vi "XW_Tutu_Chevray_PN.vi"() -> (5 "Plug in titles":string[](array[string]), 7 "Plug in values":string[](array[string]))   [LabVIEW 2020]
uses:
  Globals/Meas_global.vi
  Controls/Analysis_type_Enum.ctl
  <vilib>/Utility/file.llb/Read From Spreadsheet File (string).vi
panel:
  out "UW":bool
  out "Converged":bool=TRUE
  out "Third":dbl format="%#.3f"
  out "Filename":string
  out "Third Component":path
  out "Info index":i32
  out "2nd Comp":string
  out "1st Comp":string
  out "Psi 2":dbl=-999.0 format="%.2f"
  out "Psi 1":dbl=-999.0 format="%.2f"
  out "Indicies":i32[](array[numeric])
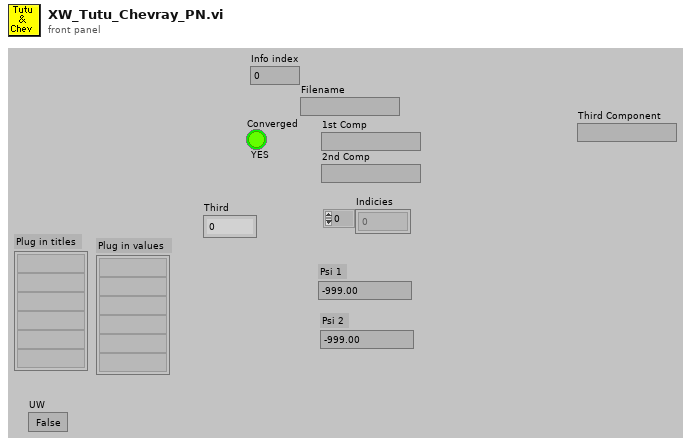
[diagram p1: front panel]
types:
  T1 = typedef "Correlation_cluster1.ctl" = cluster{"U inst":string, "uw":dbl, "u^2w":dbl, "uw^2":dbl, "uw/u'w'":dbl, "W inst":string, "uw^3":dbl, "u^3w":dbl, "u^2w^2":dbl, "Index U":i32, "Index W":i32, "Error info":string[], "Paired Sampling Rate (Hz)":dbl, "u^2 Paired":dbl, "w^2 Paired":dbl, "Time Window (ms)":dbl}
  T2 = typedef "Analysis_info_cluster.ctl" = cluster{"Colour":u32, "Inst type":T3, "Inst name":string, "Symbol":string, "Code name":string, "Extra Info":string, "Inst Array":T4, "Extra Titles":string[], "Extra Values":string[], "U":dbl, "u^2":dbl, "u^3":dbl, "u^4":dbl, "Skew_u":dbl, "Kurt_u":dbl, "Sd Error in Mean":dbl, "% u'/U":dbl, "X":dbl, "Y":dbl, "Z":dbl, "Timescale integral Estimate":dbl, "Sd Error in Variance":dbl, "Calib File":path, "Calib Constants":dbl[], "Output Position":bool, "Stats":enum16{"None", "Basic", "Full"}, "Av Sampling Rate":dbl, "Av No of Samples":dbl, "Total Meas Time (s)":dbl, "ADAM Ch Name":string, "Max value":dbl, "Min value":dbl, "Req Sample Rate Hz":dbl, "Sync Delay Time (s)":dbl, "Ch No":i16, "Device":string, "Use Latest Calib":bool, "Port":string, "Metadata Ch Names":string[], "Metadata Ch Values":string[], "Label":string}
  T3 = typedef "Inst_type.ctl" = enum16{"Raw voltage", "Raw with zero offsetting", "Propeller anemometer", "Pressure Transducer", "Pitot-static tube", "Hot wire", "Cross wire 1", "Cross wire 2", "Generic Linear", "Generic Polynomial", "Generic BackPoly", "Fast FID", "Thermocouple", "Cold wire", "Pulsed Wire", "LDA Vel", "LDA Tran time", "LDA Arr time", "Microphone"}
  T4 = typedef "Instrument_Array.ctl" = enum16{"PWA", "LDA", "Analogue"}
  T5 = typedef "Analysis_type_Enum.ctl" = enum16{"Slow Response", "Fast Response", "Weighted Fast Response", "Fast FID", "Weighted Fast FID", "Cross Wire", "Weighted Cross Wire", "Weighted LDA"}
  T6 = enum16{"Save no data", "Save data in new files", "Save data in existing files"}
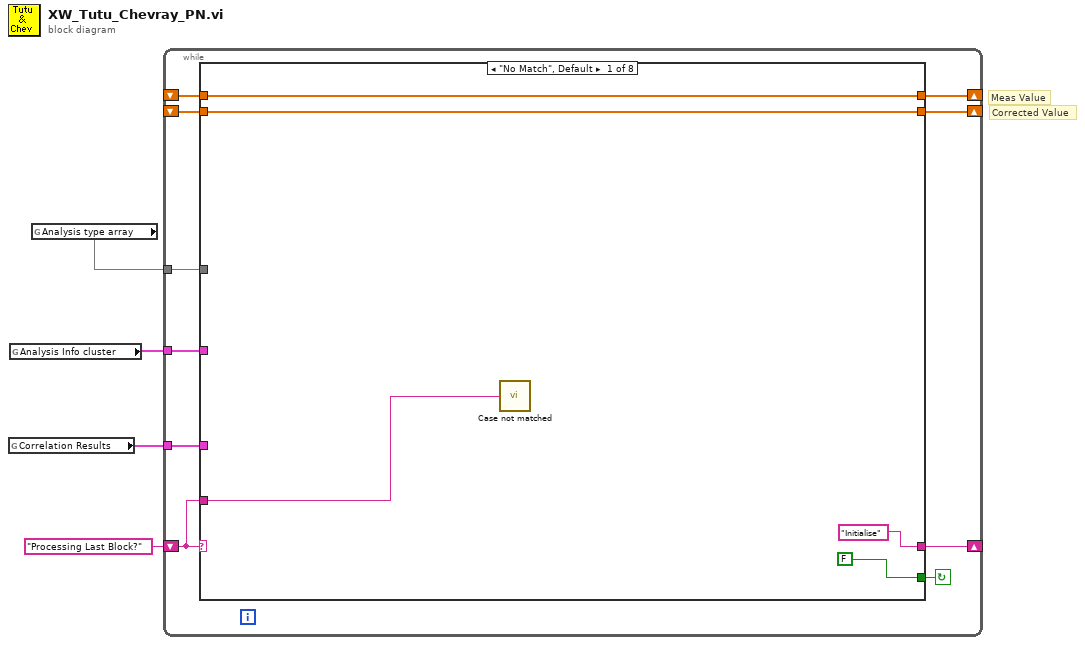
[diagram p0: block diagram]
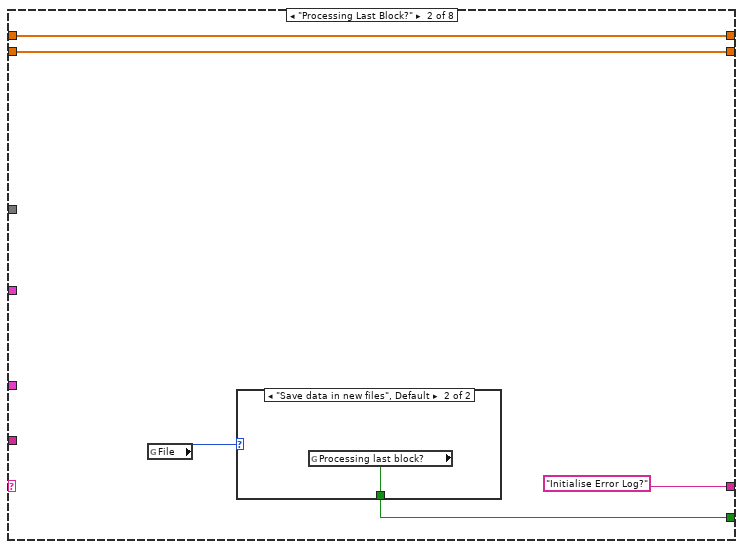
[diagram p2: hidden frame]
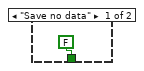
[diagram p3: hidden frame]
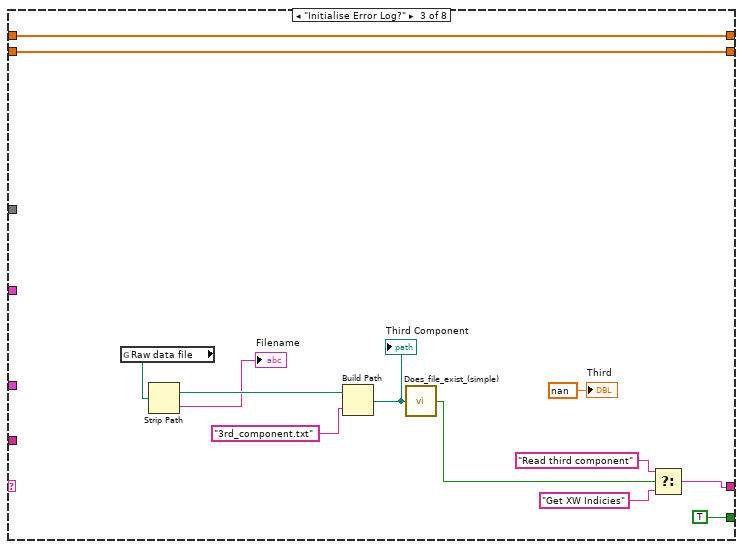
[diagram p4: hidden frame]
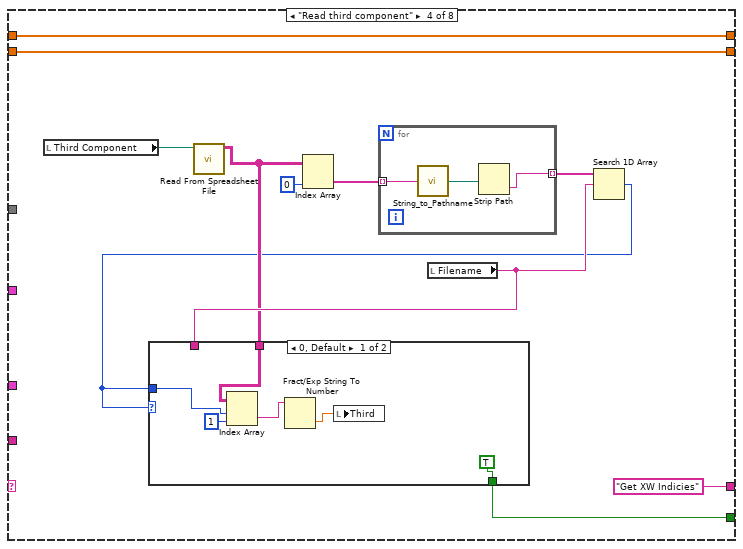
[diagram p5: hidden frame]
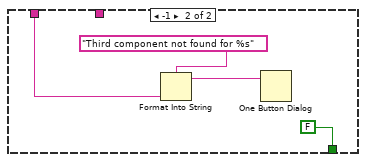
[diagram p6: hidden frame]
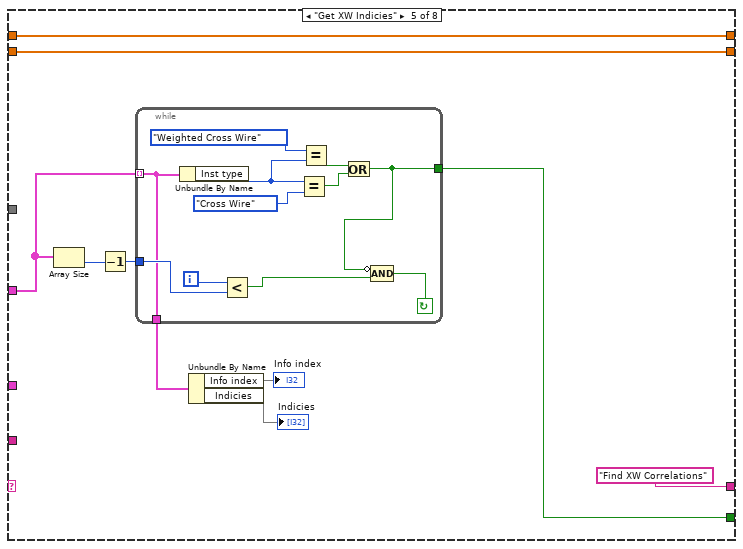
[diagram p7: hidden frame]
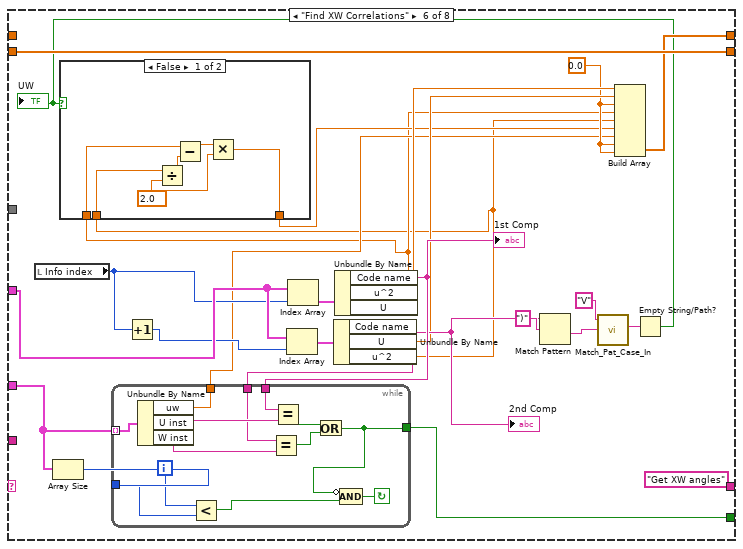
[diagram p8: hidden frame]
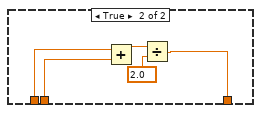
[diagram p9: hidden frame]
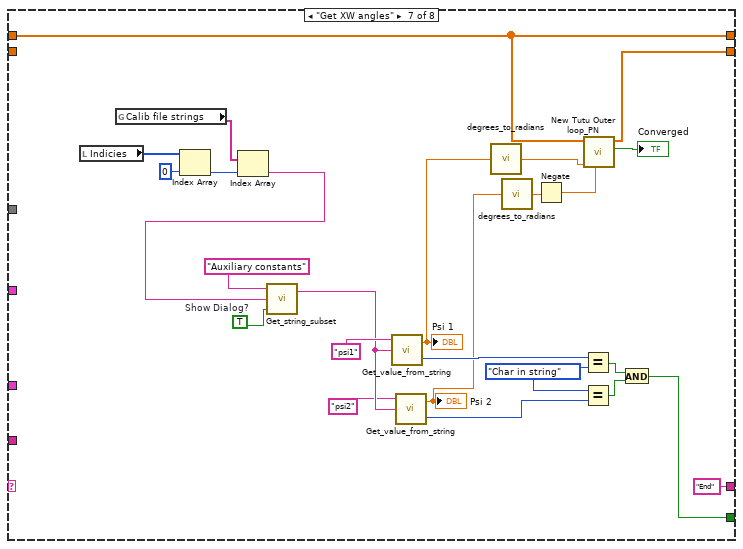
[diagram p10: hidden frame]
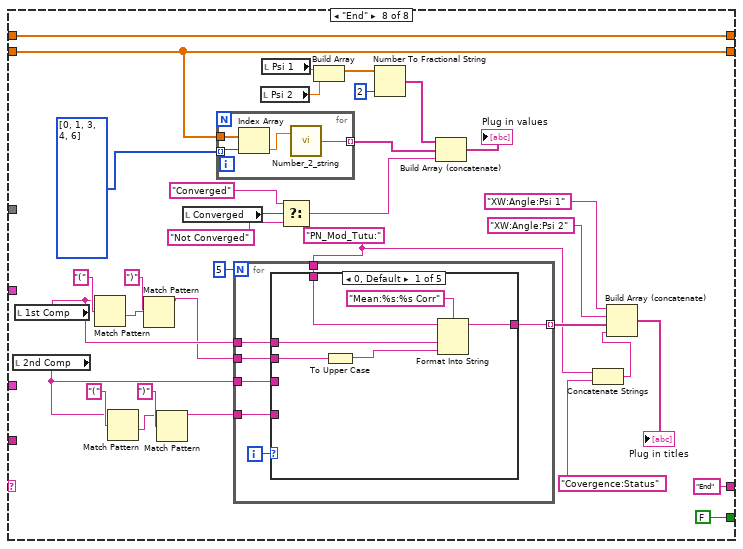
[diagram p11: hidden frame]
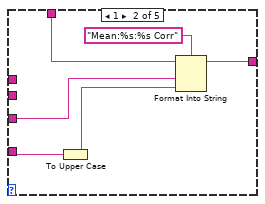
[diagram p12: hidden frame]
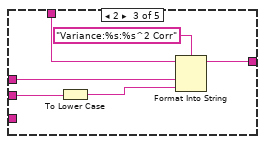
[diagram p13: hidden frame]
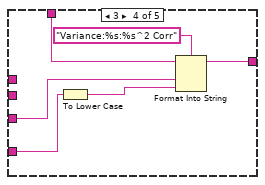
[diagram p14: hidden frame]
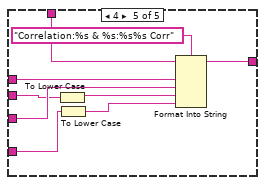
[diagram p15: hidden frame]
diagram:
  # "Corrected Value"
  # "Meas Value"
  n1 = global read "Meas_global.vi" "Correlation Results"() -> (w1:T1[])
  n2 = global read "Meas_global.vi" "Analysis Info cluster"() -> (w2:T2[])
  n3 = global read "Meas_global.vi" "Analysis type array"() -> (w3)
  n4 = while {
    tunnel: w1 -> [w6]
    tunnel: w2 -> [w7]
    tunnel: w3 -> [w11]
    shift-left: _ -> [w5]
    shift-right: [w8] -> _
    shift-left: _ -> [w9]
    shift-right: [w10] -> _
    shift-left: "Processing Last Block?" -> [w12]
    shift-right: [w13] -> _
    stop <- w14 continue-if-true
    n5 = case shown="\"No Match\", Default" w12 {
      tunnel: [FALSE w23 TRUE ("Processing last block?") w42 w69 w94 w142 FALSE ("Processing last block?")] -> w14
      tunnel: ["Initialise" "Initialise Error Log?" w29 "Get XW Indicies" "Find XW Correlations" "Get XW angles" "End" "End"] -> w13
      tunnel: w12 -> [w15 _ _ _ _ _ _ _]
      tunnel: w11 -> [_ _ _ _ _ _ _ _]
      tunnel: [w17 w22 w39 w50 w68 w96 w141 w190] -> w10
      tunnel: w9 -> [w17 w22 w39 w50 w68 _ w141 w190]
      tunnel: [w16 w20 w38 w49 w67 w108 w140 w166] -> w8
      tunnel: w7 -> [_ _ _ _ w64 w105 _ _]
      tunnel: w6 -> [_ _ _ _ _ w104 _ _]
      tunnel: w5 -> [w16 w20 w38 w49 w67 w108 _ w166]
      frame "No Match", Default {
        n6 = call "Case not matched.vi"("Case Name not Matched"=w15) -> ()
      }
      frame "Processing Last Block?" {
        n7 = global read "Meas_global.vi" "File"() -> (w21:T6)
        n8 = case shown="\"Save data in new files\", Default" w21 {
          tunnel: [FALSE ("Processing last block?") w26] -> w23
          frame "Save no data" {
          }
          frame "Save data in new files", Default {
            n9 = global read "Meas_global.vi" "Processing last block?"() -> (w26:bool)
          }
        }
      }
      frame "Initialise Error Log?" {
        n10 = global read "Meas_global.vi" "Raw data file"() -> (w36:path)
        n11 = Strip Path(path=w36) -> (stripped path=w35:path, name=→"Filename":string)
        n12 = Build Path(base path=w35, name or relative path="3rd_component.txt") -> (appended path=w33:path)
        "Third Component" <- w33
        n13 = call "Does_file_exist_(simple).vi"("Pathname"=w33) -> ("exists?"=w30:bool)
        n14 = Select(t="Read third component", s=w30, f="Get XW Indicies") -> (s? t:f=w29:string)
        "Third" <- nan ("Third")
      }
      frame "Read third component" {
        n15 = local read "Third Component"() -> (w47:path)
        n16 = call-poly <vilib>:"Read From Spreadsheet File.vi"("file path (dialog if empty)"=w47) -> ("all rows"=w41:string[][])  [unwired: 3 in, 7 out]
        n17 = Index Array(array=w41, index (col)=0 ("disabled index (col)")) -> (element=w45:string[])  [unwired: 1 in]
        n18 = for {
          tunnel: w45 -> [w63] mode=indexing
          tunnel: [w61] -> w44 mode=indexing
          n19 = call "String_to_Pathname.vi"("Input String"=w63) -> ("path"=w62:path)
          n20 = Strip Path(path=w62) -> (name=w61:string)  [unwired: 1 out]
        }
        n21 = local read "Filename"() -> (w43:string)
        n22 = Search 1D Array(1D array=w44, element=w43) -> (index of element=w40:i32)  [unwired: 1 out]
        n23 = case shown="0, Default" w40 {
          tunnel: w43 -> [_ w60]
          tunnel: [TRUE ("Processing last block?") FALSE ("Processing last block?")] -> w42
          tunnel: w41 -> [w54 _]
          tunnel: w40 -> [w53 _]
          frame 0, Default {
            n24 = Index Array(array=w54, index (row)=w53, index (col)=1 ("disabled index (col)")) -> (element=w52:string)
            n25 = Fract/Exp String To Number(string=w52) -> (number=w51:dbl)  [unwired: 4 out]
            n26 = local write "Third"(w51) -> ()
          }
          frame -1 {
            n27 = Format Into String(format string="Third component not found for %s" ("message"), w60) -> (resulting string=w58:string)  [unwired: 2 in, 1 out]
            n28 = One Button Dialog(message=w58) -> ()  [unwired: 2 out]
          }
        }
      }
      frame "Get XW Indicies" {
        n29 = Array Size(array=w64) -> (size(s)=w72:i32)
        n30 = Decrement(x=w72) -> (x-1=w71:i32)
        n31 = while {
          tunnel: [w74] -> w69
          tunnel: [w75] -> w70
          tunnel: w71 -> [w78]
          tunnel: w64 -> [w75] mode=indexing
          i -> [w79]
          stop <- w76 continue-if-true
          n32 = Unbundle By Name(w75) -> ("Inst type"=w83:T3)
          n33 = Less?(x=w79, y=w78) -> (x < y?=w77:bool)
          n34 = Equal?(x=w83, y=Analysis_type_Enum."Cross Wire" ("Analysis type")) -> (x = y?=w81:bool)
          n35 = Equal?(x=Analysis_type_Enum."Weighted Cross Wire" ("Analysis type"), y=w83) -> (x = y?=w80:bool)
          n36 = Or(x=w80, y=w81) -> (x .or. y?=w74:bool)
          n37 = Compound Arithmetic op=AND(invert w74, w77) -> (w76:bool)
        }
        n38 = Unbundle By Name(w70) -> ("Info index"=→"Info index", "Indicies"=→"Indicies")
      }
      frame "Find XW Correlations" {
        w90 = 0.0 ("element")
        n39 = local read "Info index"() -> (w93:i32)
        n40 = Array Size(array=w104) -> (size(s)=w102:i32)
        n41 = Increment(x=w93) -> (x+1=w92:i32)
        n42 = Index Array(array=w105, index=w92) -> (element=w106:T2)
        n43 = Index Array(array=w105, index=w93) -> (element=w107:T2)
        n44 = Unbundle By Name(w106) -> ("Code name"=w100:string, "U"=w91:dbl, "u^2"=w86:dbl)
        "2nd Comp" <- w100
        n45 = Unbundle By Name(w107) -> ("Code name"=w103:string, "u^2"=w87:dbl, "U"=w95:dbl)
        "1st Comp" <- w103
        n46 = while {
          tunnel: [w121] -> w89
          tunnel: w100 -> [w122]
          tunnel: w103 -> [w123]
          tunnel: w104 -> [w126] mode=indexing
          tunnel: [w127] -> w94
          tunnel: w102 -> [w130]
          i -> [w131]
          stop <- w128 continue-if-true
          n47 = Unbundle By Name(w126) -> ("uw"=w121:dbl, "U inst"=w125:string, "W inst"=w124:string)
          n48 = Less?(x=w131, y=w130) -> (x < y?=w129:bool)
          n49 = Equal?(x=w122, y=w124) -> (x = y?=w133:bool)
          n50 = Equal?(x=w123, y=w125) -> (x = y?=w132:bool)
          n51 = Or(x=w132, y=w133) -> (x .or. y?=w127:bool)
          n52 = Compound Arithmetic op=AND(invert w127, w129) -> (w128:bool)
        }
        n53 = Match Pattern(string=w100, regular expression=")") -> (after substring=w98:string)  [unwired: 4 out]
        n54 = call "Match_Pat_Case_In.vi"("String to match"="V" ("regular expression"), "String"=w98) -> ("Matched string"=w97:string)  [unwired: 1 in, 3 out]
        n55 = Empty String/Path?(string/path=w97) -> (empty?=w85:bool)
        "UW" <- w85
        n56 = case shown="False" w85 {
          tunnel: w87 -> [w111 w117]
          tunnel: w86 -> [w110 w116]
          tunnel: [w112 w118] -> w88
          frame False {
            w113 = 2.0 ("y")
            n57 = Divide(x=w110, y=w113) -> (x/y=w115:dbl)
            n58 = Subtract(x=w111, y=w115) -> (x-y=w114:dbl)
            n59 = Multiply(x=w114, y=w113) -> (x*y=w112:dbl)
          }
          frame True {
            n60 = Add(x=w117, y=w116) -> (x+y=w120:dbl)
            n61 = Divide(x=w120, y=2.0) -> (x/y=w118:dbl)
          }
        }
        n62 = Build Array(w95, w91, w90, w87, w86, w88, w89, w90, w90) -> (w96:dbl[])
      }
      frame "Get XW angles" {
        w147 = enum16{"Char in string", "Char not in string"}."Char in string" ("Status")
        w153 = TRUE  # Show Dialog?
        n63 = local read "Indicies"() -> (w157:i32[])
        n64 = global read "Meas_global.vi" "Calib file strings"() -> (w156:string[])
        n65 = Index Array(array=w157, index=0 ("Index")) -> (element=w155:i32)
        n66 = Index Array(array=w156, index=w155) -> (element=w152:string)
        n67 = call "Get_string_subset.vi"("Show Dialog?"=w153, "String to split"=w152, "File Label"="Auxiliary constants") -> ("Output string"=w150:string)  [unwired: 1 in, 1 out]
        n68 = call "Get_value_from_string.vi"("Input string"=w150, "Variable name"="psi1") -> ("Status"=w146:enum16{"Char in string", "Char not in string"}, "Value"=w134:dbl)  [unwired: 1 in]
        "Psi 1" <- w134
        n69 = call "Get_value_from_string.vi"("Input string"=w150, "Variable name"="psi2") -> ("Status"=w145:enum16{"Char in string", "Char not in string"}, "Value"=w138:dbl)  [unwired: 1 in]
        "Psi 2" <- w138
        n70 = call "degrees_to_radians.vi"("degrees"=w134) -> ("radians"=w135:dbl)
        n71 = call "degrees_to_radians.vi"("degrees"=w138) -> ("radians"=w137:dbl)
        n72 = Negate(x=w137) -> (-x=w136:dbl)
        n73 = Equal?(x=w146, y=w147) -> (x = y?=w143:bool)
        n74 = Equal?(x=w147, y=w145) -> (x = y?=w144:bool)
        n75 = call "New Tutu Outer loop_PN.vi"("Const psi2"=w136, "Const psi1"=w135, "Measured stats"=w141) -> ("Converged"=→"Converged":bool, "Corrected stats"=w140:dbl[])  [unwired: 7 out]
        n76 = And(x=w143, y=w144) -> (x .and. y?=w142:bool)
      }
      frame "End" {
        w160 = "PN_Mod_Tutu:"
        n77 = local read "2nd Comp"() -> (w179:string)
        n78 = local read "1st Comp"() -> (w183:string)
        n79 = Match Pattern(string=w183, regular expression="(") -> (after substring=w188:string)  [unwired: 4 out]
        n80 = Match Pattern(string=w179, regular expression="(") -> (after substring=w184:string)  [unwired: 4 out]
        n81 = Match Pattern(string=w188, regular expression=")") -> (before substring=w182:string)  [unwired: 4 out]
        n82 = Match Pattern(string=w184, regular expression=")") -> (before substring=w178:string)  [unwired: 4 out]
        n83 = local read "Converged"() -> (w165:bool)
        n84 = for {
          tunnel: [w196] -> w168 mode=indexing
          tunnel: i32[] [0, 1, 3, 4, 6] -> [w195] mode=indexing
          tunnel: w166 -> [w193]
          n85 = Index Array(array=w193, index=w195) -> (element=w194:dbl)
          n86 = call "Number_2_string.vi"("number"=w194) -> ("String"=w196:string)  [unwired: 1 in]
        }
        n87 = for {
          N: 5 -> [_]
          tunnel: w160 -> [w202]
          tunnel: w183 -> [w201]
          tunnel: w182 -> [w200]
          tunnel: [w199] -> w181 mode=indexing
          tunnel: w179 -> [w198]
          tunnel: w178 -> [w197]
          i -> [w203]
          n88 = case shown="0, Default" w203 {
            tunnel: w202 -> [w204 w212 w216 w222 w228]
            tunnel: w201 -> [w206 _ w220 _ w233]
            tunnel: w200 -> [w208 _ w218 _ w231]
            tunnel: [w205 w213 w219 w226 w235] -> w199
            tunnel: w198 -> [_ w210 _ w224 w232]
            tunnel: w197 -> [_ w211 _ w223 w234]
            frame 0, Default {
              n89 = To Upper Case(1:w208) -> (0:w209:string)
              n90 = Format Into String(format string="Mean:%s:%s Corr" ("Format String"), initial string=w204, w206, w209) -> (resulting string=w205:string)  [unwired: 1 in, 1 out]
            }
            frame 1 {
              n91 = To Upper Case(1:w211) -> (0:w215:string)
              n92 = Format Into String(format string="Mean:%s:%s Corr" ("Format String"), initial string=w212, w210, w215) -> (resulting string=w213:string)  [unwired: 1 in, 1 out]
            }
            frame 2 {
              n93 = To Lower Case(string=w218) -> (all lower case string=w217:string)
              n94 = Format Into String(format string="Variance:%s:%s^2 Corr" ("Format String"), initial string=w216, w220, w217) -> (resulting string=w219:string)  [unwired: 1 in, 1 out]
            }
            frame 3 {
              n95 = To Lower Case(string=w223) -> (all lower case string=w225:string)
              n96 = Format Into String(format string="Variance:%s:%s^2 Corr" ("Format String"), initial string=w222, w224, w225) -> (resulting string=w226:string)  [unwired: 1 in, 1 out]
            }
            frame 4 {
              n97 = To Lower Case(string=w231) -> (all lower case string=w230:string)
              n98 = To Lower Case(string=w234) -> (all lower case string=w229:string)
              n99 = Format Into String(format string="Correlation:%s & %s:%s%s Corr" ("Format String"), initial string=w228, w233, w232, w230, w229) -> (resulting string=w235:string)  [unwired: 1 in, 1 out]
            }
          }
        }
        n100 = local read "Psi 2"() -> (w171:dbl)
        n101 = local read "Psi 1"() -> (w172:dbl)
        n102 = Select(t="Converged", s=w165, f="Not Converged") -> (s? t:f=w162:string)
        n103 = Build Array(w172, w171) -> (w170:dbl[])
        n104 = Number To Fractional String(number=w170, precision (6)=i16 2) -> (F-format string=w169:string[])  [unwired: 2 out]
        n105 = Build Array (concatenate)(w169, w168, w162) -> (→"Plug in values":string[])
        n106 = Concatenate Strings(w160, "Covergence:Status" ("string")) -> (w161:string)
        n107 = Build Array (concatenate)("XW:Angle:Psi 1", "XW:Angle:Psi 2", w181, w161) -> (→"Plug in titles":string[])
      }
    }
  }
